vi "Draw_Line.vi"(6 "Error in (no error)":errorcluster, 8 "All balls \ncoordinates":T3(array[cluster]), 10 "BillardBox":T1, 11 "Image data":T2) -> (3 "New picture":picture, 4 "Error out":errorcluster)   [LabVIEW 2019]
doc: "Draw_Line.vi\nDraw the billard box and trajectory of each ball on PNG file.\nInput : -BillardBox containing the coordinates of the billard box\n -All balls coordinates (array of Balls coordinates) containing coordinates and score of each balls from the begining of the sequence.\n -Image data containing information of PNG file\n -Error in\nOutput : -New picture with trajectory and billard box in overprint on PNG\n -Error out"
uses:
  <vilib>/picture/picture.llb/imagedata.ctl
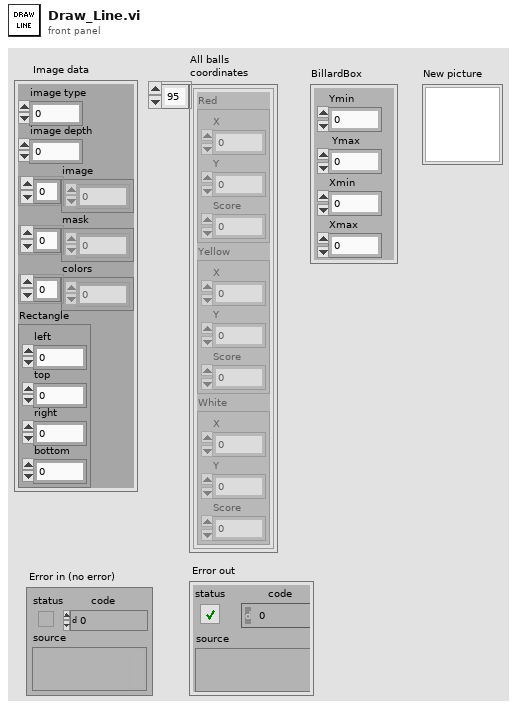
[diagram p1: front panel]
types:
  T1 = cluster{"Ymin":dbl, " Ymax":dbl, "Xmin":dbl, "Xmax":dbl}
  T2 = typedef "imagedata.ctl" = cluster{"image type":i32, "image depth":i32, "image":u8[], "mask":u8[], "colors":u32[], "Rectangle":cluster{"left":i16, "top":i16, "right":i16, "bottom":i16}}
  T3 = cluster{"Red":cluster{"X":dbl, "Y":dbl, "Score":dbl}, "Yellow":cluster{"X":dbl, "Y":dbl, "Score":dbl}, "White":cluster{"X":dbl, "Y":dbl, "Score":dbl}}[]
  T4 = cluster{"Xmin":dbl, "Ymin":dbl, "Xmax":dbl, " Ymax":dbl}
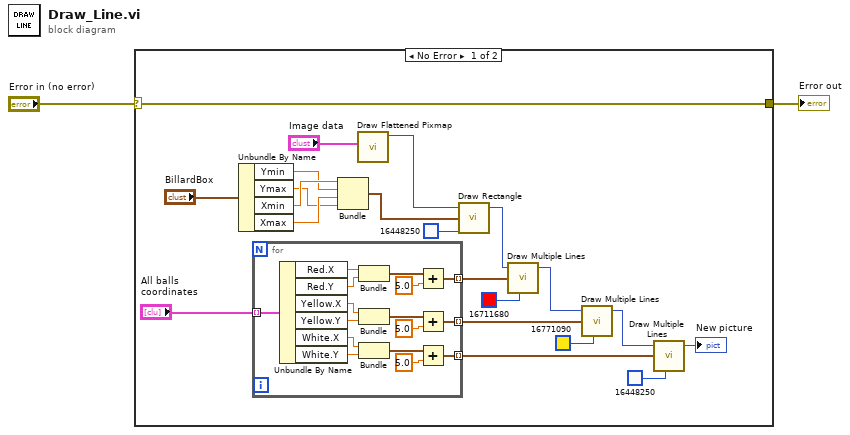
[diagram p0: block diagram]
diagram:
  n1 = case shown="No Error" "Error in (no error)" {
    selector: "Error in (no error)" -> [w3 w40]
    tunnel: [w3 w40] -> w1
    frame No Error {
      n2 = Unbundle By Name("BillardBox") -> ("Ymin"=w6:dbl, "Ymax"=w4:dbl, "Xmin"=w7:dbl, "Xmax"=w5:dbl)
      n3 = for {
        tunnel: "All balls \ncoordinates" -> [w33] mode=indexing
        tunnel: [w26] -> w16 mode=indexing
        tunnel: [w25] -> w15 mode=indexing
        tunnel: [w24] -> w14 mode=indexing
        n4 = Unbundle By Name(w33) -> ("Red.X"=w39:dbl, "Red.Y"=w38:dbl, "Yellow.X"=w37:dbl, "Yellow.Y"=w36:dbl, "White.X"=w35:dbl, "White.Y"=w34:dbl)
        n5 = Bundle("X"=w39, "Y"=w38) -> (w29:cluster{"X":dbl, "Y":dbl})  [unwired: 1 in]
        n6 = Bundle("X"=w37, "Y"=w36) -> (w28:cluster{"X":dbl, "Y":dbl})  [unwired: 1 in]
        n7 = Bundle("X"=w35, "Y"=w34) -> (w27:cluster{"X":dbl, "Y":dbl})  [unwired: 1 in]
        n8 = Add(x=w29, y=5.0) -> (x+y=w26:cluster{"X":dbl, "Y":dbl})
        n9 = Add(x=w28, y=5.0) -> (x+y=w25:cluster{"X":dbl, "Y":dbl})
        n10 = Add(x=w27, y=5.0) -> (x+y=w24:cluster{"X":dbl, "Y":dbl})
      }
      n11 = Bundle("Xmin"=w7, "Ymin"=w6, "Xmax"=w5, "Ymax"=w4) -> (w8:T4)  [unwired: 1 in]
      n12 = call <vilib>:"Draw Flattened Pixmap.vi"("image data"="Image data") -> ("new picture"=w9:picture)  [unwired: 8 in]
      n13 = call <vilib>:"Draw Rectangle.vi"("picture"=w9, "rect"=w8, "color(black)"=u32 16448250) -> ("new picture"=w10:picture)  [unwired: 6 in]
      n14 = call <vilib>:"Draw Multiple Lines.vi"("picture"=w10, "line endpoints"=w16, "color(black)"=u32 16711680) -> ("new picture"=w22:picture)  [unwired: 6 in]
      n15 = call <vilib>:"Draw Multiple Lines.vi"("picture"=w22, "line endpoints"=w15, "color(black)"=u32 16771090) -> ("new picture"=w21:picture)  [unwired: 6 in]
      n16 = call <vilib>:"Draw Multiple Lines.vi"("picture"=w21, "line endpoints"=w14, "color(black)"=u32 16448250) -> ("new picture"=→"New picture":picture)  [unwired: 6 in]
    }
    frame Error {
    }
  }
  "Error out" <- w1
